vi "onHeartbeat.vi"(8 "error in (no error)":errorcluster, 10 "model in":refnum<class "IModel.lvclass">, 11 "EnabledState in":refnum<class "EnabledState.lvclass">) -> (0 "error out":errorcluster, 2 "model out":refnum<class "IModel.lvclass">, 3 "EnabledState out":refnum<class "EnabledState.lvclass">)   [LabVIEW 2012, in "States.lvlib" / "EnabledState.lvclass"]
uses:
  EnabledState.lvclass
  IModel/IModel.lvclass
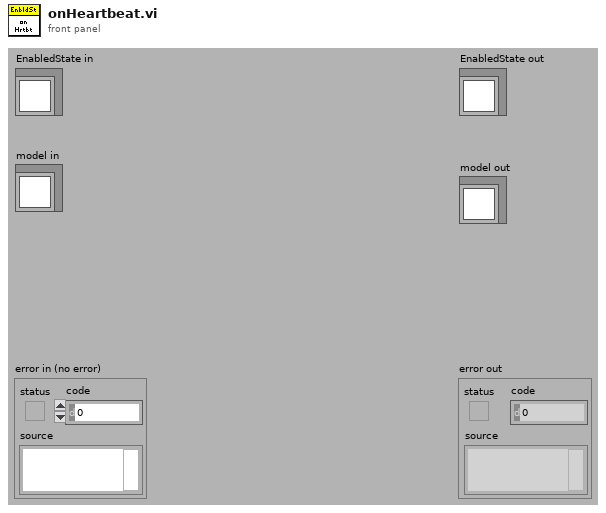
[diagram p1: front panel]
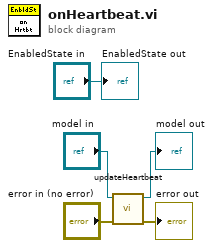
[diagram p0: block diagram]
diagram:
  n1 = call-dynamic "updateHeartbeat.vi"("error in (no error)"="error in (no error)", "IModel in"="model in") -> ("error out"=→"error out":errorcluster, "IModel out"=→"model out":refnum<class "IModel.lvclass">)  [unwired: 7 in, 1 out]
  "EnabledState out" <- "EnabledState in"
